vi "unregisterEvents.vi"(8 "error in (no error)":errorcluster, 11 "SAL_Listener in":refnum<class "SAL_Listener.lvclass">) -> (0 "error out":errorcluster, 3 "SAL_Listener out":refnum<class "SAL_Listener.lvclass">)   [LabVIEW 2015, in "SAL_Listener.lvclass"]
uses:
  SAL_Listener.lvclass
  SALLV_dome/SALLV_dome.lvlib
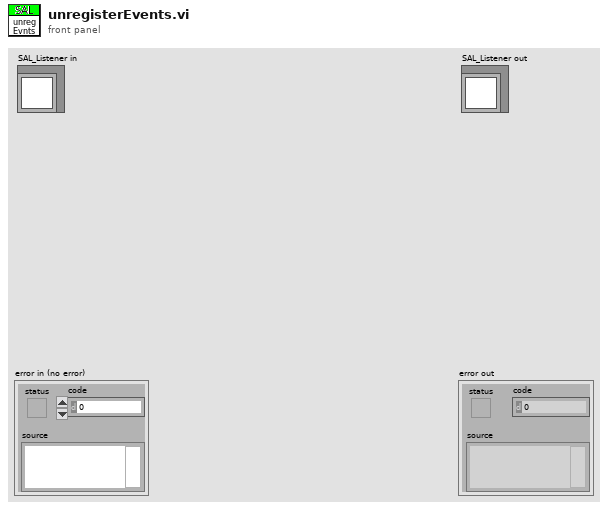
[diagram p1: front panel]
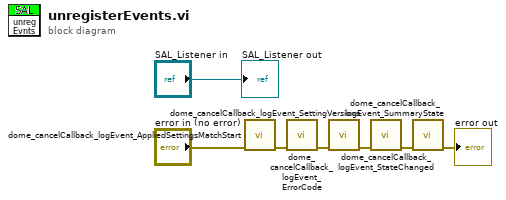
[diagram p0: block diagram]
diagram:
  n1 = call "dome_cancelCallback_logEvent_AppliedSettingsMatchStart.vi"("error in (no error)"="error in (no error)") -> ("error out"=w6:errorcluster)  [unwired: 9 in, 1 out]
  n2 = call "dome_cancelCallback_logEvent_ErrorCode.vi"("error in (no error)"=w6) -> ("error out"=w5:errorcluster)  [unwired: 9 in, 1 out]
  n3 = call "dome_cancelCallback_logEvent_SettingVersions.vi"("error in (no error)"=w5) -> ("error out"=w4:errorcluster)  [unwired: 9 in, 1 out]
  n4 = call "dome_cancelCallback_logEvent_StateChanged.vi"("error in (no error)"=w4) -> ("error out"=w3:errorcluster)  [unwired: 9 in, 1 out]
  n5 = call "dome_cancelCallback_logEvent_SummaryState.vi"("error in (no error)"=w3) -> ("error out"=→"error out":errorcluster)  [unwired: 9 in, 1 out]
  "SAL_Listener out" <- "SAL_Listener in"
